vi "progra 5.vi"() -> ()   [LabVIEW 2011]
panel:
  out "Personas":dbl
  in  "Planta":u16(ring) items=["Planta #1", "planta #2", "Planta #3"]
  out "A/c":bool
  out "Temperatura":i32(slide) scale=0.0..60.0
  # "Se genera la temperatura entre 1-60,\nse selecciona la planta usando el menu ring,\nluego se genera el numero de personas entre 1-50"
  # "Planta 1 si hay mas de 25 personas y la temperatura \nes mayor a 25 se enciende el A/C\n\nPlanta 2 si hay ma de 30 personas la y la temperatura\nes mayot a 27 se enciende el A/C\n\nPlanta 3 si hay ma de 20 personas la y la temperatura\nes mayor a 28 se enciende el A/C"
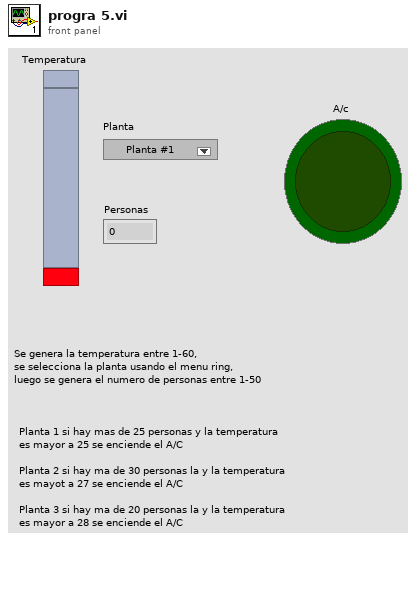
[diagram p1: front panel]
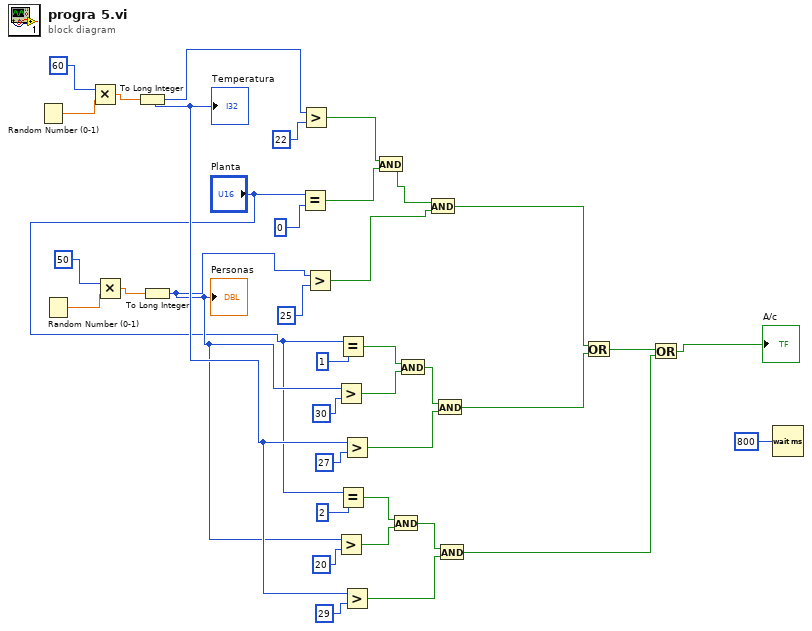
[diagram p0: block diagram]
diagram:
  n1 = Random Number (0-1)() -> (number: 0 to 1=w36:dbl)
  n2 = Random Number (0-1)() -> (number: 0 to 1=w31:dbl)
  n3 = Multiply(x=60, y=w36) -> (x*y=w35:dbl)
  n4 = Multiply(x=50, y=w31) -> (x*y=w32:dbl)
  n5 = To Long Integer(number=w35) -> (32bit integer=w13:i32)
  "Temperatura" <- w13
  n6 = To Long Integer(number=w32) -> (32bit integer=w12:i32)
  "Personas" <- w12
  n7 = Equal?(x="Planta", y=0) -> (x = y?=w26:bool)
  n8 = Greater?(x=w13, y=22) -> (0:w27:bool)
  n9 = Greater?(x=w12, y=25) -> (0:w24:bool)
  n10 = Greater?(x=w12, y=30) -> (0:w19:bool)
  n11 = Greater?(x=w12, y=20) -> (0:w10:bool)
  n12 = Equal?(x="Planta", y=1) -> (x = y?=w20:bool)
  n13 = Equal?(x="Planta", y=2) -> (x = y?=w11:bool)
  n14 = Greater?(x=w13, y=27) -> (0:w17:bool)
  n15 = Greater?(x=w13, y=29) -> (0:w8:bool)
  n16 = And(x=w27, y=w26) -> (x .and. y?=w25:bool)
  n17 = And(x=w11, y=w10) -> (x .and. y?=w9:bool)
  n18 = And(x=w20, y=w19) -> (x .and. y?=w18:bool)
  n19 = And(x=w25, y=w24) -> (x .and. y?=w7:bool)
  n20 = And(x=w18, y=w17) -> (x .and. y?=w6:bool)
  n21 = And(x=w9, y=w8) -> (x .and. y?=w4:bool)
  n22 = Or(x=w7, y=w6) -> (x .or. y?=w5:bool)
  n23 = Or(x=w5, y=w4) -> (x .or. y?=→"A/c":bool)
  n24 = Wait (ms)(milliseconds to wait=800) -> ()  [unwired: 1 out]
